vi "Ustaw obiekty rejestracja.vi"(7 "WaveformGraph in":refnum<vi>, 8 "error in (no error)":errorcluster, 10 "Bounds":T1, 11 "Array":refnum<vi>[](array[refnum])) -> (0 "error out":errorcluster, 2 "Rejestracja Bounds":T1[](array[typedef]))   [LabVIEW 2014]
doc: "Pozycjonuje położenie obiektów w zakładce Rejestracja"
uses:
  <vilib>/Utility/miscctls.llb/LVBoundsTypeDef.ctl
  <vilib>/Utility/miscctls.llb/LVPositionTypeDef.ctl
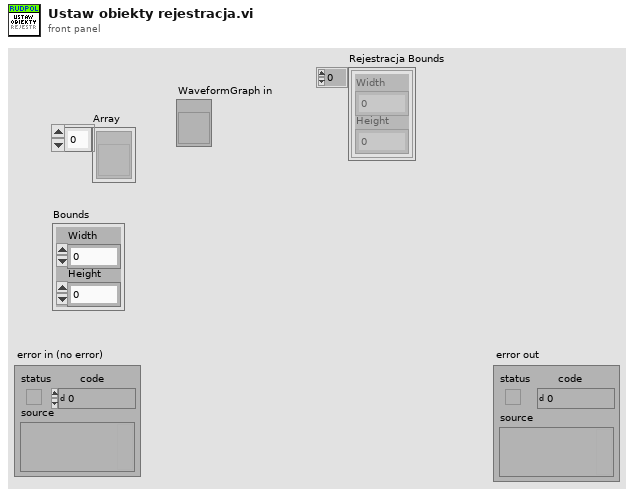
[diagram p1: front panel]
types:
  T1 = typedef "LVBoundsTypeDef.ctl" = cluster{"Width":u32, "Height":u32}
  T2 = typedef "LVPositionTypeDef.ctl" = cluster{"Left":i32, "Top":i32}
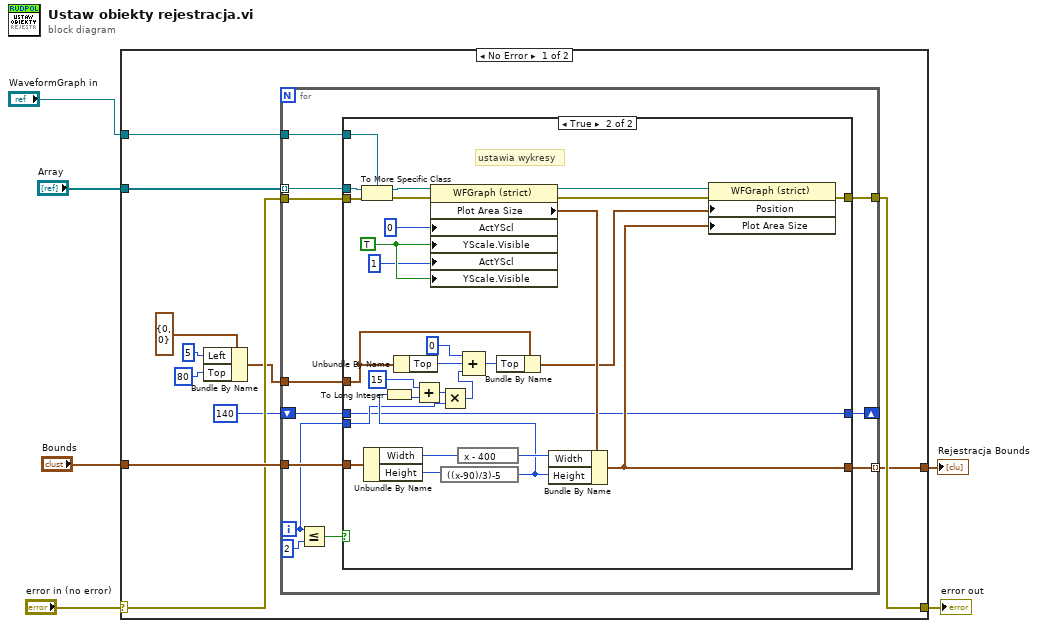
[diagram p0: block diagram]
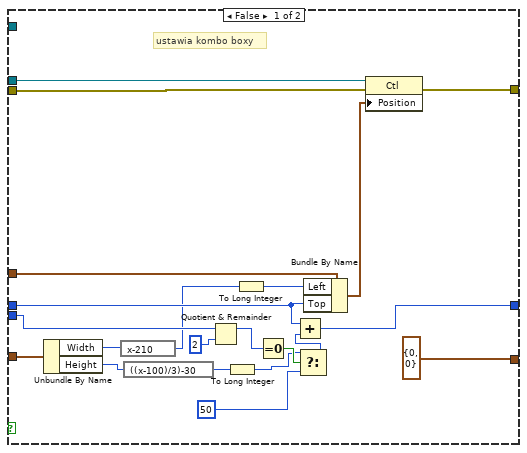
[diagram p2: hidden frame]
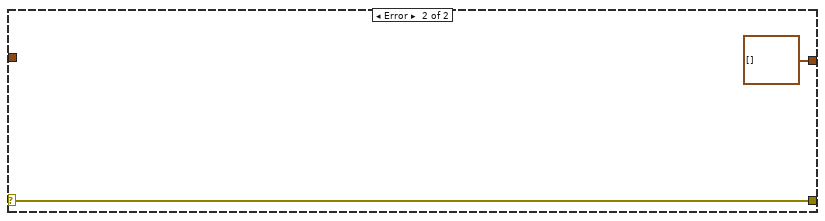
[diagram p3: hidden frame]
diagram:
  n1 = case shown="No Error" "error in (no error)" {
    selector: "error in (no error)" -> [w14 w81]
    tunnel: [w13 w81] -> w5
    tunnel: "Array" -> [w17 _]
    tunnel: "Bounds" -> [w16 _]
    tunnel: "WaveformGraph in" -> [w15 _]
    tunnel: [w9 T1[] []] -> w1
    frame No Error {
      n2 = Bundle By Name(cluster=T2 {"Left"=0, "Top"=0} ("Position"), "Left"=5 ("y"), "Top"=80 ("y")) -> (w8:T2)
      n3 = for {
        tunnel: w17 -> [w27] mode=indexing
        tunnel: w16 -> [w26]
        tunnel: w15 -> [w25]
        tunnel: w14 -> [w24]
        tunnel: [w23] -> w13
        tunnel: [w21] -> w9 mode=indexing
        tunnel: w8 -> [w20]
        shift-right: [w19] -> _
        shift-left: 140 ("Top") -> [w18]
        i -> [w22]
        n4 = Less Or Equal?(x=w22, y=2) -> (x <= y?=w28:bool)
        n5 = case shown="True" w28 {
          tunnel: w27 -> [w46 w79]
          tunnel: w26 -> [w45 w67]
          tunnel: w25 -> [_ w78]
          tunnel: w24 -> [w47 w77]
          tunnel: [w48 w76] -> w23
          tunnel: w22 -> [w39 w58]
          tunnel: [T1 {"Width"=0, "Height"=0} ("Plot Area Size") w63] -> w21
          tunnel: w20 -> [w49 w60]
          tunnel: [w41 w54] -> w19
          tunnel: w18 -> [w42 w54]
          frame False {
            # "ustawia kombo boxy"
            n6 = Unbundle By Name(w45) -> ("Width"=w44:u32, "Height"=w40:u32)
            n7 = expression code="x-210"(w44) -> (w32:u32)
            n8 = expression code="((x-100)/3)-30"(w40) -> (w31:u32)
            n9 = Quotient & Remainder(x=w39, y=2) -> (x-y*floor(x/y)=w37:i32)  [unwired: 1 out]
            n10 = To Long Integer(number=w31) -> (32bit integer=w30:i32)
            n11 = To Long Integer(number=w32) -> (32bit integer=w33:i32)
            n12 = Equal To 0?(x=w37) -> (x = 0?=w36:bool)
            n13 = Select(t=w30, s=w36, f=50 ("y")) -> (s? t:f=w34:i32)
            n14 = Add(x=w42, y=w34) -> (x+y=w41:i32)
            n15 = Bundle By Name(cluster=w49, "Left"=w33, "Top"=w42) -> (w43:T2)
            n16 = property class="Ctl"(reference=w46, error in=w47, "Position"=w43) -> (error out=w48:errorcluster)  [unwired: 1 out]
          }
          frame True {
            w53 = TRUE ("Y Scale.Visible")
            # "ustawia wykresy"
            n17 = To More Specific Class(target class=w78, reference=w79, error in=w77) -> (specific class reference=w74:refnum<vi>, error out=w75:errorcluster)
            n18 = Unbundle By Name(w67) -> ("Width"=w69:u32, "Height"=w68:u32)
            n19 = Unbundle By Name(w60) -> ("Top"=w64:i32)
            n20 = property class="WFGraph (strict)"(reference=w74, error in=w75, "ActYScl"=0 ("Active Y Scale"), "YScale.Visible"=w53, "ActYScl"=1 ("Active Y Scale"), "YScale.Visible"=w53) -> (reference out=w72:refnum<vi>, error out=w73:errorcluster, "Plot Area Size"=w71:T1)
            n21 = expression code="((x-90)/3)-5"(w68) -> (w62:u32)
            n22 = To Long Integer(number=w62) -> (32bit integer=w57:i32)
            n23 = Add(x=15 ("value"), y=w57) -> (x+y=w56:i32)
            n24 = Multiply(x=w56, y=w58) -> (x*y=w59:i32)
            n25 = expression code="x - 400"(w69) -> (w70:u32)
            n26 = Compound Arithmetic op=ADD(0 ("value"), w64, w59) -> (w66:i32)
            n27 = Bundle By Name(cluster=w60, "Top"=w66) -> (w61:T2)
            n28 = Bundle By Name(cluster=w71, "Width"=w70, "Height"=w62) -> (w63:T1)
            n29 = property class="WFGraph (strict)"(reference=w72, error in=w73, "Position"=w61, "Plot Area Size"=w63) -> (error out=w76:errorcluster)  [unwired: 1 out]
          }
        }
      }
    }
    frame Error {
    }
  }
  "error out" <- w5
  "Rejestracja Bounds" <- w1
